vi "construct.vi"(8 "error in (no error)":errorcluster, 9 "configuration name":string, 10 "load config file?":bool=TRUE, 11 "GenericPlugin in":refnum<class "ScanHeadAK130114ResonanceFlexRIO.lvclass">) -> (0 "error out":errorcluster, 3 "GenericPlugin out":refnum<class "ScanHeadAK130114ResonanceFlexRIO.lvclass">)   [LabVIEW 2010, in "ScanHeadAK130114ResonanceFlexRIO.lvclass"]
uses:
  ScanHeadAK130114ResonanceFlexRIO.lvclass
  GenericScanHead/GenericScanHead/GenericScanHead.lvclass
  ScanHeadAK130114ResonanceFlexRIO.lvclass/ScanHeadAK130114ResonanceFlexRIO.ctl
  SignalWriter/GenericSignalWriter/GenericSignalWriter/GenericSignalWriter.lvclass
  AnalogOut/GenericAnalogOut/GenericAnalogOut/GenericAnalogOut.lvclass
  common/classes/ErrorController/ErrorController/class_data.vi
  common/classes/GenericComponent/GenericComponent/GenericComponent.lvclass
  common/classes/ErrorController/ErrorController/ErrorController.lvclass
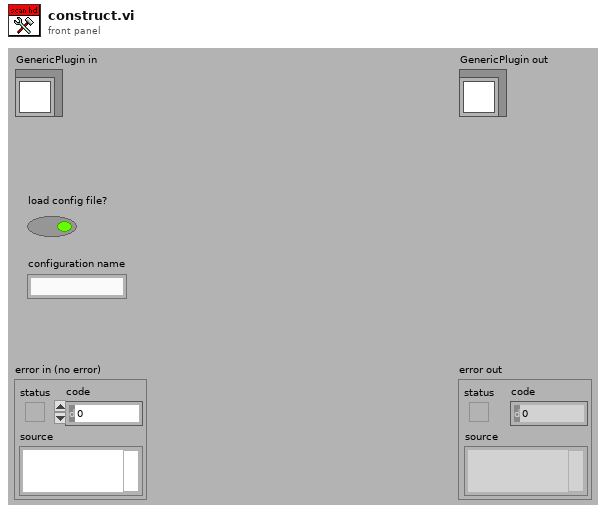
[diagram p1: front panel]
types:
  T1 = typedef "plugin_specification.ctl" = cluster{"class path":string, "configuration":string, "label":string, "settings name":string}
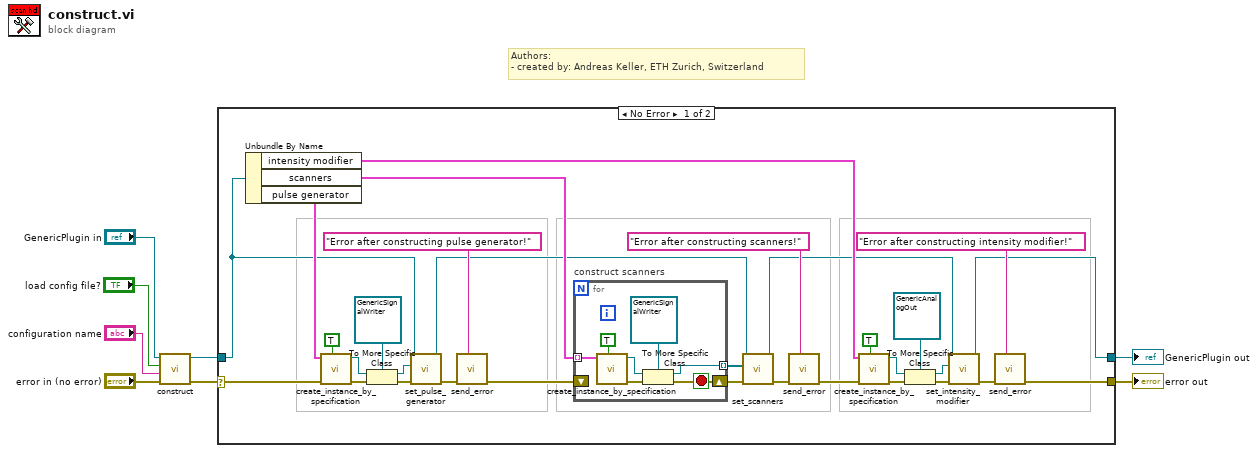
[diagram p0: block diagram]
diagram:
  # "Authors: \n- created by: Andreas Keller, ETH Zurich, Switzerland"
  n1 = call-parent "construct.vi"("error in (no error)"="error in (no error)", "configuration name"="configuration name", "load config file?"="load config file?", "GenericPlugin in"="GenericPlugin in") -> ("error out"=w4:errorcluster, "GenericPlugin out"=w2:refnum<class "ScanHeadAK130114ResonanceFlexRIO.lvclass">)  [unwired: 6 in]
  n2 = case shown="No Error" w4 {
    selector: w4 -> [w38 w48]
    tunnel: [w15 w48] -> w3
    tunnel: [w9 w47] -> w1
    tunnel: w2 -> [w12 w47]
    frame No Error {
      n3 = Unbundle By Name(w12) -> ("intensity modifier"=w13:T1, "scanners"=w23:T1[], "pulse generator"=w39:T1)
      n4 = call "create_instance_by_specification.vi"("call constructor?"=TRUE, "error in (no error)"=w38, "component specification"=w39) -> ("error out"=w37:errorcluster, "GenericPlugin out"=w36:refnum<class "GenericComponent.lvclass">)  [unwired: 6 in, 1 out]
      n5 = To More Specific Class(target class=refnum<class "GenericSignalWriter.lvclass"> refnum ("pulse generator"), reference=w36, error in=w37) -> (specific class reference=w33:refnum<class "GenericSignalWriter.lvclass">, error out=w35:errorcluster)
      n6 = call-dynamic "set_pulse_generator.vi"("error in (no error)"=w35, "pulse generator"=w33, "ScanHeadAK130114ResonanceFlexRIO in"=w12) -> ("error out"=w32:errorcluster, "ScanHeadAK130114ResonanceFlexRIO out"=w11:refnum<class "ScanHeadAK130114ResonanceFlexRIO.lvclass">)  [unwired: 7 in]
      n7 = call "send_error.vi"("additional message"="Error after constructing pulse generator!", "error in (no error)"=w32) -> ("error out"=w22:errorcluster)  [unwired: 9 in]
      n8 = for "construct scanners" {
        tunnel: w23 -> [w42] mode=indexing
        shift-right: [w41] -> w21
        shift-left: w22 -> [_]
        tunnel: [w40] -> w20 mode=indexing
        stop <- w41 stop-if-true
        n9 = call "create_instance_by_specification.vi"("call constructor?"=TRUE, "component specification"=w42) -> ("error out"=w46:errorcluster, "GenericPlugin out"=w45:refnum<class "GenericComponent.lvclass">)  [unwired: 7 in, 1 out]
        n10 = To More Specific Class(target class=refnum<class "GenericSignalWriter.lvclass"> refnum ("pulse generator"), reference=w45, error in=w46) -> (specific class reference=w40:refnum<class "GenericSignalWriter.lvclass">, error out=w41:errorcluster)
      }
      n11 = call-dynamic "set_scanners.vi"("error in (no error)"=w21, "scanners"=w20, "ScanHeadAK130114ResonanceFlexRIO in"=w11) -> ("error out"=w28:errorcluster, "ScanHeadAK130114ResonanceFlexRIO out"=w10:refnum<class "ScanHeadAK130114ResonanceFlexRIO.lvclass">)  [unwired: 7 in]
      n12 = call "send_error.vi"("additional message"="Error after constructing scanners!", "error in (no error)"=w28) -> ("error out"=w14:errorcluster)  [unwired: 9 in]
      n13 = call "create_instance_by_specification.vi"("call constructor?"=TRUE, "error in (no error)"=w14, "component specification"=w13) -> ("error out"=w27:errorcluster, "GenericPlugin out"=w26:refnum<class "GenericComponent.lvclass">)  [unwired: 6 in, 1 out]
      n14 = To More Specific Class(target class=refnum<class "GenericAnalogOut.lvclass"> refnum ("GenericAnalogOut.lvclass"), reference=w26, error in=w27) -> (specific class reference=w17:refnum<class "GenericAnalogOut.lvclass">, error out=w18:errorcluster)
      n15 = call-dynamic "set_intensity_modifier.vi"("error in (no error)"=w18, "intensity modifier"=w17, "ScanHeadAK130114ResonanceFlexRIO in"=w10) -> ("error out"=w16:errorcluster, "ScanHeadAK130114ResonanceFlexRIO out"=w9:refnum<class "ScanHeadAK130114ResonanceFlexRIO.lvclass">)  [unwired: 7 in]
      n16 = call "send_error.vi"("additional message"="Error after constructing intensity modifier!", "error in (no error)"=w16) -> ("error out"=w15:errorcluster)  [unwired: 9 in]
    }
    frame Error {
    }
  }
  "error out" <- w3
  "GenericPlugin out" <- w1
